vi "Create Test Configuration.vi"() -> (0 "error out":errorcluster, 1 "Names":string[](array[string]), 2 "Line Array":T1[](array[typedef]), 3 "Module Configuration":refnum<class "tag bus configurable plugin module configuration.lvclass">, 4 "Channels":refnum<class "TBM channel.lvclass">[](array[class]), 5 "instance identifier":string)   [LabVIEW 2014, in "io plugin tests.lvlib"]
doc: "This VI creates a standard test configuration for other unit tests. It currently creates and adds one line with every datatype to the module configuration."
uses:
  module/configuration/tag bus configurable plugin module configuration.lvclass
  module/configuration/Line.ctl
  <vilib>/NI/Tag Bus Module Framework/channel/TBM channel.lvclass
  <vilib>/NI/Tag Bus Module Framework/channel/channel classification.ctl
  io plugin tests.lvlib
  <vilib>/NI/Configuration Framework/serializable configuration/NISE_CEF_serializable configuration.lvclass
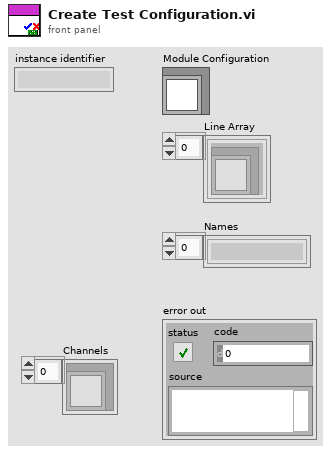
[diagram p1: front panel]
types:
  T1 = typedef "tag bus configurable plugin module configuration.lvclass/Line.ctl" = cluster{"channel":refnum<class "TBM channel.lvclass">}
  T2 = typedef "TBM channel.lvclass/channel classification.ctl" = enum16{"input data", "output data", "processing parameter", "processing result"}
  T3 = typedef "tag bus.lvlib/tag descriptor.lvclass/Data Type.ctl" = enum16{"Double", "Single", "I64", "I32", "I16", "I8", "U64", "U32", "U16", "U8", "Boolean", "String", "Array of Double", "Array of Single", "Array of I64", "Array of I32", "Array of I16", "Array of I8", "Array of U64", "Array of U32", "Array of U16", "Array of U8", "Array of Boolean", "Array of String"}
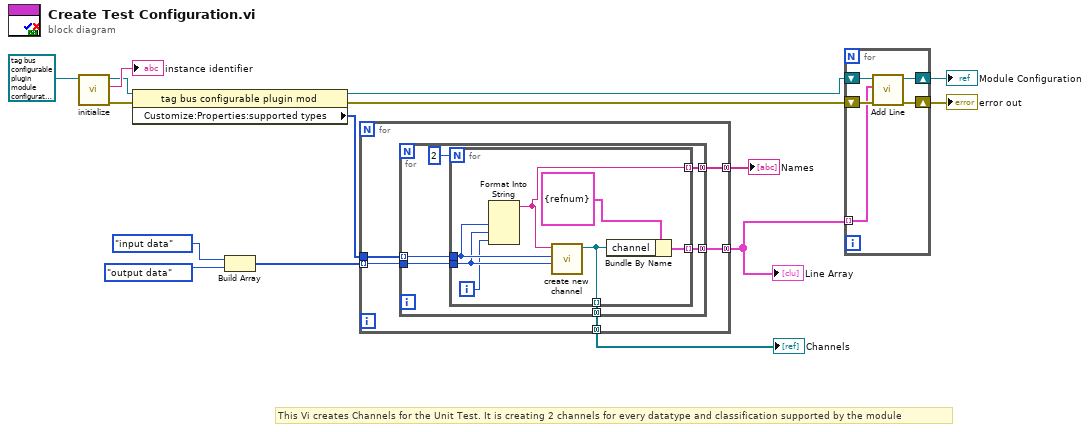
[diagram p0: block diagram]
diagram:
  # "This Vi creates Channels for the Unit Test. It is creating 2 channels for every datatype and classification supported by the module"
  n1 = call <vilib>:"initialize.vi"("configuration in"=refnum<class "tag bus configurable plugin module configuration.lvclass"> refnum ("tag bus configurable plugin module configuration")) -> ("error out"=w13:errorcluster, "identifier"=→"instance identifier":string, "configuration out"=w10:refnum<class "tag bus configurable plugin module configuration.lvclass">)  [unwired: 8 in]
  n2 = property class="tag bus configurable plugin mod"(reference=w10, error in=w13) -> (reference out=w5:refnum<class "tag bus configurable plugin module configuration.lvclass">, error out=w12:errorcluster, "Customize:Properties:supported types"=w6:T3[])
  n3 = Build Array(channel_classification."input data" ("channel classification"), channel_classification."output data" ("channel classification")) -> (w4:T2[])
  n4 = for {
    tunnel: w4 -> [w20] mode=indexing
    tunnel: [w18] -> w9 mode=concatenating
    tunnel: w6 -> [w19]
    tunnel: [w17] -> w11 mode=concatenating
    tunnel: [w16] -> w1 mode=concatenating
    n5 = for {
      tunnel: w20 -> [w26]
      tunnel: [w24] -> w18 mode=concatenating
      tunnel: w19 -> [w25] mode=indexing
      tunnel: [w22] -> w17 mode=concatenating
      tunnel: [w23] -> w16 mode=concatenating
      n6 = for {
        N: 2 -> [_]
        tunnel: w26 -> [w30]
        tunnel: w25 -> [w31]
        tunnel: [w27] -> w24 mode=indexing
        tunnel: [w32] -> w23 mode=indexing
        tunnel: [w28] -> w22 mode=indexing
        i -> [w29]
        n7 = Format Into String(w31, w30, w29) -> (resulting string=w28:string)  [unwired: 3 in, 1 out]
        n8 = call <vilib>:"create new channel.vi"("channel classification"=w30, "data type"=w31, "channel name"=w28) -> ("channel"=w32:refnum<class "TBM channel.lvclass">)  [unwired: 8 in]
        n9 = Bundle By Name(cluster=T1 {"channel"=refnum} ("Line"), "channel"=w32) -> (w27:T1)
      }
    }
  }
  "Names" <- w11
  "Line Array" <- w9
  "Channels" <- w1
  n10 = for {
    tunnel: w9 -> [w34] mode=indexing
    shift-right: [w37] -> w8
    shift-left: w5 -> [w38]
    shift-right: [w35] -> w15
    shift-left: w12 -> [w36]
    n11 = call "Add Line.vi"("error in"=w36, "Line"=w34, "tag bus configurable plugin module configuration in"=w38) -> ("error out"=w35:errorcluster, "tag bus configurable plugin module configuration out"=w37:refnum<class "tag bus configurable plugin module configuration.lvclass">)  [unwired: 6 in, 1 out]
  }
  "error out" <- w15
  "Module Configuration" <- w8
